vi "Validate Configuration (Transfer).vi"(8 "error in (no error)":errorcluster, 11 "transfer configuration in":T1 {"channel blocks"."string descriptor"."buffer offset" format="%d bytes"; "channel blocks"."engine descriptor"."buffer offset" format="%d bytes"}) -> (0 "error out":errorcluster, 3 "transfer configuration out":T1 {"channel blocks"."string descriptor"."buffer offset" format="%d bytes"; "channel blocks"."engine descriptor"."buffer offset" format="%d bytes"})   [LabVIEW 2017, in "DSF Core.lvlib"]
uses:
  DSF Core.lvlib
  Controls/DSF Engine Transfer Configuration.ctl
  Controls/DSF Byte Order.ctl
  Controls/DSF Engine Channel Configuration.ctl
  Controls/DSF Channel Buffer Descriptor.ctl
  Controls/DSF Data Type.ctl
  Controls/DSF Settings Info.ctl
  Shared/VIs/Sizeof 1D.vi
  Errors/Errors.vi
  Errors/Channel Overlap.vi
  Shared/VIs/Sizeof.vi
  Errors/New Configuration Error.vi
  <vilib>/NI/Memory Manager/VIs/Source.Write.String.vi
  <vilib>/NI/Memory Manager/VIs/Source.Write.Scalar.Base10.vi
  <vilib>/NI/Memory Manager/VIs/Source.Write.Scalar.Base10 (U64).vi
  Shared/Constants/Constants.vi
  Shared/Constants/Engine Library Name.vi
  <vilib>/NI/Memory Manager/VIs/Error Cluster.Set VI Source.vi
  <vilib>/NI/Memory Manager/VIs/Error Cluster.Set Code.vi
  <vilib>/NI/Memory Manager/VIs/Error Cluster.Set Status.vi
  <vilib>/NI/Memory Manager/VIs/New Error Cluster Constant.vi
  <vilib>/NI/Memory Manager/VIs/New Error Cluster Constant (512B).vi
  Errors/Configuration Error Info.vi
  Shared/Constants/Base Error Code.vi
  Shared/Constants/Error Offset (Configuration).vi
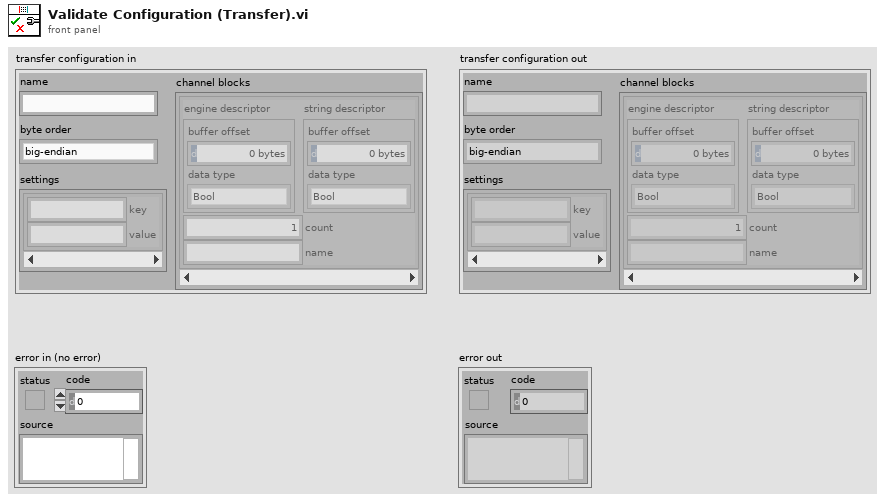
[diagram p1: front panel]
types:
  T1 = typedef "DSF Core.lvlib/DSF Engine Transfer Configuration.ctl" = cluster{"name":string, "byte order":T2, "channel blocks":T3[], "settings":T6}
  T2 = typedef "DSF Core.lvlib/DSF Byte Order.ctl" = enum8{"big-endian", "little-endian"}
  T3 = typedef "DSF Core.lvlib/DSF Engine Channel Configuration.ctl" = cluster{"engine descriptor":T4, "string descriptor":T4, "count":u64, "name":string}
  T4 = typedef "DSF Core.lvlib/DSF Channel Buffer Descriptor.ctl" = cluster{"buffer offset":u64, "data type":T5}
  T5 = typedef "DSF Core.lvlib/DSF Data Type.ctl" = enum8{"Bool", "SGL", "DBL", "I8", "I16", "I32", "I64", "U8", "U16", "U32", "U64"}
  T6 = typedef "DSF Core.lvlib/DSF Settings Info.ctl" = cluster{"key":string, "value":string}[]
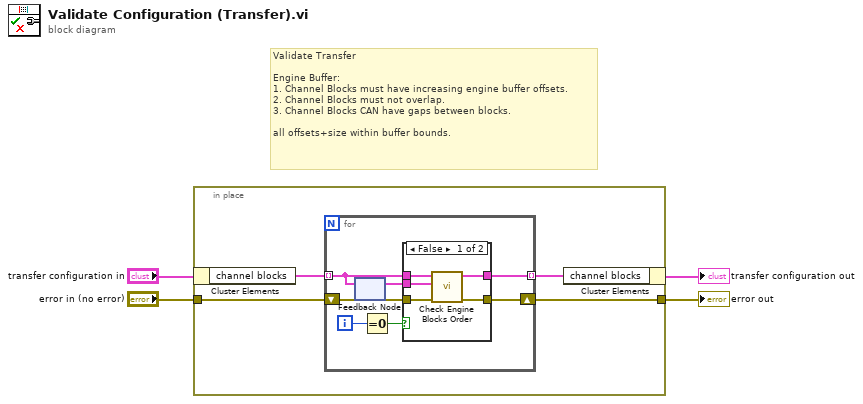
[diagram p0: block diagram]
diagram:
  # "Validate Transfer\n\nEngine Buffer:\n1. Channel Blocks must have increasing engine buffer offsets.\n2. Channel Blocks must not overlap.\n3. Channel Blocks CAN have gaps between blocks.\n\nall offsets+size within buffer bounds."
  n1 = in-place {
    in-place-border: [w8] -> w4
    in-place-border: "error in (no error)" -> [w7]
    n2 = in-place-cluster #1("transfer configuration in") -> ("channel blocks"=w6:T3[])
    n3 = for {
      tunnel: w6 -> [w13] mode=indexing
      tunnel: [w11] -> w5 mode=indexing
      shift-right: [w10] -> w8
      shift-left: w7 -> [w9]
      i -> [w15]
      n4 = feedback #2() -> (w12:T3)  [unwired: 1 in]
      n5 = feedback-in #2(w13) -> ()
      n6 = Equal To 0?(x=w15) -> (x = 0?=w14:bool)
      n7 = case shown="False" w14 {
        tunnel: w13 -> [w17 w21]
        tunnel: [w17 w21] -> w11
        tunnel: w12 -> [w19 _]
        tunnel: [w16 w20] -> w10
        tunnel: w9 -> [w18 w20]
        frame False {
          n8 = call "Check Engine Blocks Order.vi"("error in (no error)"=w18, "previous channel block"=w19, "channel block"=w17) -> ("error out"=w16:errorcluster)  [unwired: 8 in]
        }
        frame True {
        }
      }
    }
    n9 = in-place-cluster #1("channel blocks"=w5) -> (→"transfer configuration out":T1)
  }
  "error out" <- w4
